vi "TPRHOdll.vi"(8 "error in (no error)":errorcluster, 11 "Inputs":T2={"t"=0.0, "p"=0.0, "x"=[], "phase"=4, "First Guess for Rho?"=FALSE, "rho "=0.0} {"phase" items=["Liquid"=3, "Vapor"=4, "Stable Phase - Not allowed"=2, "Liquid - Metastable"=1, "Vapror - Metastable"=0]}) -> (0 "error out":errorcluster, 3 "Outputs":T1)   [LabVIEW 2016]
doc: "subroutine TPRHO (T,P,z,kph,kguess,D,ierr,herr, herr_length)\n\niterate for density as a function of temperature, pressure, and\ncomposition for a specified phase\n\n***********************************************************************\n WARNING:\n Invalid densities will be returned for T & P outside range of validity,\n i.e., pressure > melting pressure, pressure less than saturation\n pressure for kph=1, etc.\n\n***********************************************************************\nINPUTS:\nT -- temperature [K]\nP -- pressure [kPa]\nz -- composition [array of mol frac]\nkph -- 1 - Liquid phase\n 2 - Vapor phase\n 0 - Stable phase - NOT ALLOWED (use TPFLSH)\n (Unless an initial guess is supplied for D)\n -1 - Force the search in the liquid phase (for metastable points)\n -2 - Force the search in the vapor phase (for metastable points)\nkguess -- Guess flag:\n 0 - No first guess for D provided\n 1 - First guess for D provided\nD -- first guess for molar density [mol/L], only if kguess = 1\n\nOUTPUTS:\nD -- molar density [mol/L]\nierr -- error flag: 0 = successful\n 200 = CRITP did not converge\n 201 = illegal input (kph <= 0)\n 202 = liquid-phase iteration did not converge\n 203 = vapor-phase iteration did not converge\nherr -- error string (character*255 variable if ierr<>0)"
uses:
  REFPROP.DLL
panel:
  # "REFPROP-TPRHO_dll.vi"
  # "void  TPRHOdll(double *T, double *P, double *z, int32_t *kph, int32_t *kguess, double *D, int32_t *ierr, CStr herr, int32_t herr_length);"
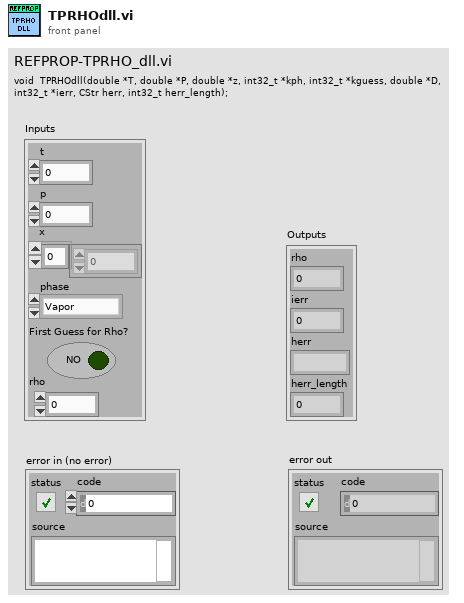
[diagram p1: front panel]
types:
  T1 = cluster{"rho":dbl, "ierr":i32, "herr":string, "herr_length":i32}
  T2 = cluster{"t":dbl, "p":dbl, "x":dbl[], "phase":u16, "First Guess for Rho?":bool, "rho ":dbl}
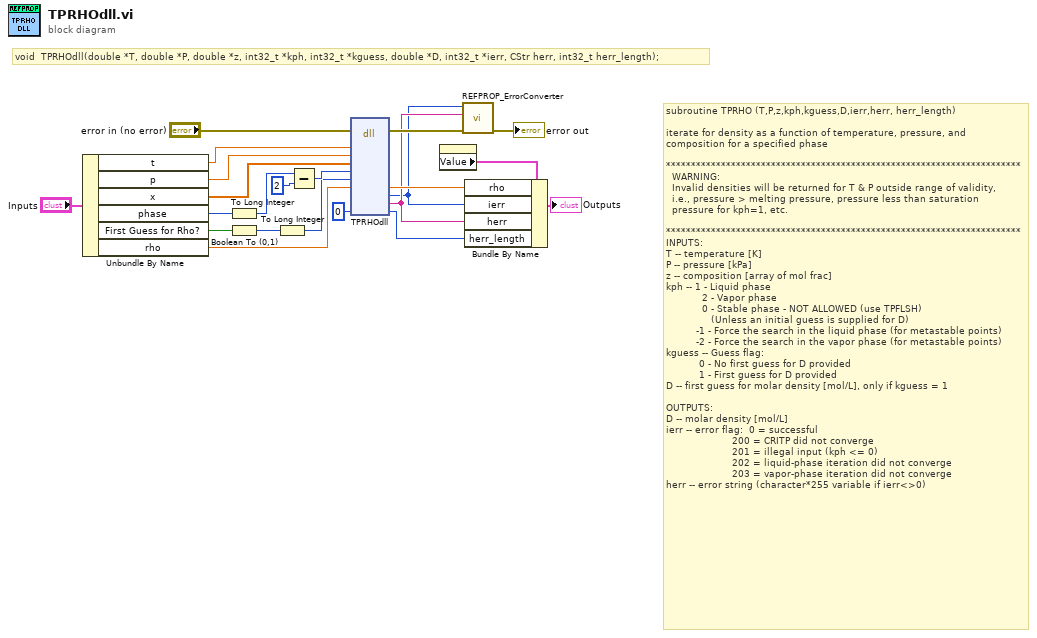
[diagram p0: block diagram]
diagram:
  # "void  TPRHOdll(double *T, double *P, double *z, int32_t *kph, int32_t *kguess, double *D, int32_t *ierr, CStr herr, int32_t herr_length);"
  # "subroutine TPRHO (T,P,z,kph,kguess,D,ierr,herr, herr_length)\n\niterate for density as a function of temperature, pressure, and\ncomposition for a specified phase\n\n***********************************************************************\n  WARNING:\n  Invalid densities will be returned for T & P outside range of validity,\n  i.e., pressure > melting pressure, pressure less than saturation\n  pressure for kph=1, etc.\n\n***********************************************************************\nINPUTS:\nT -- temperature [K]\nP -- pressure [kPa]\nz -- composition [array of mol frac]\nkph -- 1 - Liquid phase\n            2 - Vapor phase\n            0 - Stable phase - NOT ALLOWED (use TPFLSH)\n               (Unless an initial guess is supplied for D)\n          -1 - Force the search in the liquid phase (for metastable points)\n          -2 - Force the search in the vapor phase (for metastable points)\nkguess -- Guess flag:\n           0 - No first guess for D provided\n           1 - First guess for D provided\nD -- first guess for molar density [mol/L], only if kguess = 1\n\nOUTPUTS:\nD -- molar density [mol/L]\nierr -- error flag:  0 = successful\n                      200 = CRITP did not converge\n                      201 = illegal input (kph <= 0)\n                      202 = liquid-phase iteration did not converge\n                      203 = vapor-phase iteration did not converge\nherr -- error string (character*255 variable if ierr<>0)"
  n1 = Unbundle By Name("Inputs") -> ("t"=w12:dbl, "p"=w11:dbl, "x"=w10:dbl[], "phase"=w9:u16, "First Guess for Rho?"=w8:bool, "rho"=w7:dbl)
  n2 = To Long Integer(number=w9) -> (32bit integer=w18:i32)
  n3 = Boolean To (0,1)(Boolean=w8) -> (0, 1=w16:i16)
  n4 = To Long Integer(number=w16) -> (32bit integer=w14:i32)
  n5 = Subtract(x=w18, y=2) -> (x-y=w15:i32)
  n6 = dll-call lib="S:/009 - Testing/02 - Performance Testing/REFPROP/REFPROP.*" fn="TPRHOdll"(error in="error in (no error)", "T"=w12, "P"=w11, "z"=w10, "kph"=w15, "kguess"=w14, "D"=w7, "herr_length"=0 ("ln")) -> (error out=w22:errorcluster, "D"=w4:dbl, "ierr"=w1:i32, "herr"=w3:string, "herr_length"=w2:i32)  [unwired: 10 in, 1 out]
  n7 = property on="Outputs" class="Clust (strict)"() -> ("Value"=w5:T1)  [unwired: 2 in, 2 out]
  n8 = call "REFPROP_ErrorConverter.vi"("error in (no error)"=w22, "Error Message"=w3, "Error Code"=w1) -> ("error out"=→"error out":errorcluster)  [unwired: 8 in]
  n9 = Bundle By Name(cluster=w5, "rho"=w4, "ierr"=w1, "herr"=w3, "herr_length"=w2) -> (→"Outputs":T1)
